vi "MeasGroupResult.vi"(8 "error in (no error)":errorcluster, 10 "measurement_group_id":u16, 11 "ByteQXAPIBase in":refnum<class "ByteQXAPIBase.lvclass">) -> (0 "error out":errorcluster, 1 "measurements":cluster{"id":u32, "passed":bool}[](array[cluster]), 2 "measurement-group-passed":bool, 3 "ByteQXAPIBase out":refnum<class "ByteQXAPIBase.lvclass">)   [LabVIEW 2019, in "ByteQXWebAPI.lvlib" / "ByteQXAPIBase.lvclass"]
doc: "Obtain the result of the measures based on the measurement-group-id"
uses:
  ByteQXAPIBase.lvclass
  <vilib>/Bytelabs/ByteREST/ByteRESTClass/ByteRESTBase/HTTP/Status_Code.ctl
  TypeDef/Meas_Group_Res_REQ.ctl
  TypeDef/Meas_Group_Res_Data.ctl
  Private/module.ctl
  ByteQXAPIBase.lvclass/ByteQXAPIBase.ctl
  <vilib>/Bytelabs/ByteREST/ByteRESTClass/ByteRESTBase/RESTBase.lvclass
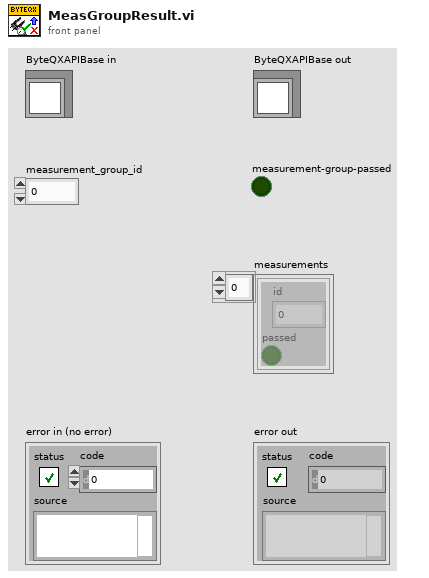
[diagram p1: front panel]
types:
  T1 = typedef "ByteQXWebAPI.lvlib/ByteQXAPIBase.lvclass/module.ctl" = enum16{"gs", "tms"}
  T2 = typedef "ByteQXWebAPI.lvlib/ByteQXAPIBase.lvclass/Meas_Group_Res_Data.ctl" = cluster{"measurement_group_passed":bool, "measurements":cluster{"id":u32, "passed":bool}[]}
  T3 = typedef "ByteQXWebAPI.lvlib/ByteQXAPIBase.lvclass/Meas_Group_Res_REQ.ctl" = cluster{"measurement_group_id":u32}
  T4 = typedef "ByteREST.lvlib/RESTBase.lvclass/Status_Code.ctl" = u16
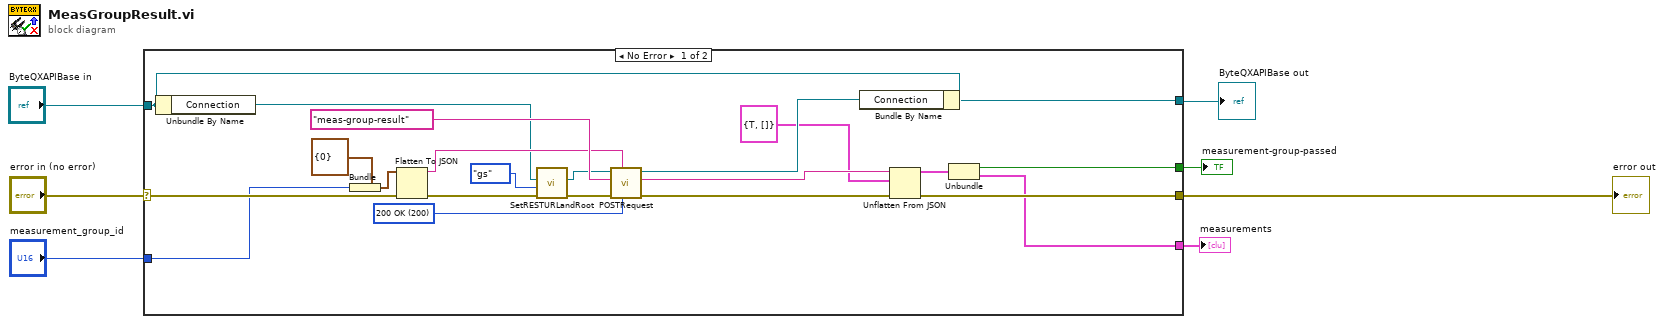
[diagram p0: block diagram]
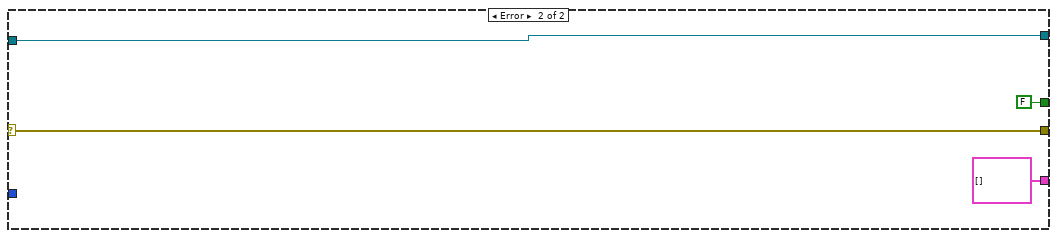
[diagram p2: hidden frame]
diagram:
  n1 = case shown="No Error" "error in (no error)" {
    selector: "error in (no error)" -> [w25 w33]
    tunnel: [w20 w33] -> w6
    tunnel: [w28 w32] -> w4
    tunnel: "ByteQXAPIBase in" -> [w29 w32]
    tunnel: "measurement_group_id" -> [w17 _]
    tunnel: [w14 FALSE ("measurement_group_passed")] -> w2
    tunnel: [w13 cluster{"id":u32, "passed":bool}[] [] ("measurements")] -> w1
    frame No Error {
      w22 = T4 200 items=["200 OK"=200, "201 Created"=201, "400 Bad Request"=400, "401 Unauthorized"=401, "403 Forbidden"=403, "404 Not Found"=404, "405 Method Not Allowed"=405, "406 Not Acceptable"=406, "500 Internal Server Error"=500] ("expected response")
      n2 = Unbundle By Name(w29) -> ("Connection"=w12:refnum<class "RESTBase.lvclass">)
      n3 = Bundle(cluster=T3 {"measurement_group_id"=0} ("MeasGroupResult_REQ"), "measurement_group_id"=w17) -> (w19:T3)
      n4 = Flatten To JSON(anything=w19, error in (no error)=w25) -> (JSON string=w21:string, 11:w9:errorcluster)  [unwired: 1 in]
      n5 = call "SetRESTURLandRoot.vi"("error in (no error)"=w9, "module"=module."gs", "ByteREST in"=w12) -> ("error out"=w8:errorcluster, "ByteREST out"=w11:refnum<class "RESTBase.lvclass">)  [unwired: 7 in]
      n6 = call-dynamic "POSTRequest.vi"("expected response"=w22, "Body in"=w21, "error in (no error)"=w8, "Request"="meas-group-result", "ByteRESTBase in"=w11) -> ("error out"=w23:errorcluster, "Body"=w24:string, "ByteRESTBase out"=w27:refnum<class "RESTBase.lvclass">)  [unwired: 3 in, 1 out]
      n7 = Bundle By Name(cluster=w29, "Connection"=w27) -> (w28:refnum<class "ByteQXAPIBase.lvclass">)
      n8 = Unflatten From JSON(JSON string=w24, type and defaults=T2 {"measurement_group_passed"=TRUE, "measurements"=[]}, error in (no error)=w23) -> (value=w18:T2, error out=w20:errorcluster)  [unwired: 4 in]
      n9 = Unbundle(w18) -> ("measurement_group_passed"=w14:bool, "measurements"=w13:cluster{"id":u32, "passed":bool}[])
    }
    frame Error {
    }
  }
  "error out" <- w6
  "ByteQXAPIBase out" <- w4
  "measurement-group-passed" <- w2
  "measurements" <- w1
